vi "MTS_GenFileComment.vi"(0 "Resolution":dbl, 1 "Measurement Type":T2(ring)=enum."Image File", 3 "Parent File No":i32=-1, 5 "Pixels":i32[](array[numeric]), 7 "Info":string, 9 "Upper Left":T4, 11 "error in":errorcluster, 12 "Time Per Pixel [ms]":dbl, 13 "Trigger":dbl[](array[numeric])) -> (4 "Comment":string, 6 "Image Info":T3, 10 "Image Header":T1, 15 "error out":errorcluster)   [LabVIEW 2013]
panel:
  in  "Scan Axis":enum32{"x-y", "x-z", "y-x", "y-z", "z-x", "z-y"}(ring)
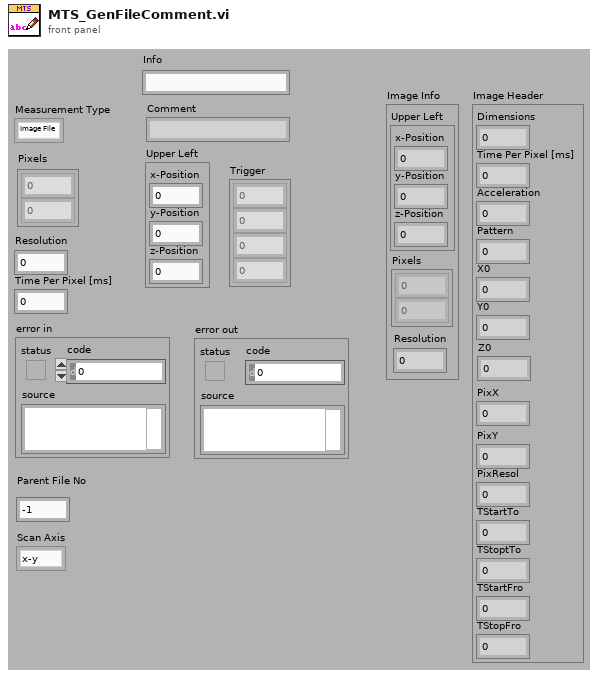
[diagram p1: front panel]
types:
  T1 = cluster{"Dimensions":i32, "Time Per Pixel [ms]":dbl, "Acceleration":i32, "Pattern":i32, "X0":sgl, "Y0":sgl, "Z0":dbl, "PixX":i32, "PixY":i32, "PixResol":sgl, "TStartTo":sgl, "TStoptTo":sgl, "TStartFro":sgl, "TStopFro":sgl}
  T2 = enum16{"not a pt3 File", "Image File", "Point Measurement", "Auto Point", "Line Scan", "Grid Scan"}
  T3 = cluster{"Upper Left":cluster{"x-Position":dbl, "y-Position":dbl, "z-Position":dbl}, "Pixels":i32[], "Resolution":dbl}
  T4 = cluster{"x-Position":dbl, "y-Position":dbl, "z-Position":dbl}
  T5 = enum16{"not a pt3 File", "Image File", "Point Measurement", "Auto Point"}
  T6 = cluster{"File No":i32, "File Path":path, "Parent File":i32, "File Type":enum16{"unknown", "pt3 File", "png Image", "bmp Image"}, "Measurement Type":enum16{"not a pt3 File", "Image File", "Point Measurement", "Auto Point", "Line Scan", "Grid Scan"}, "Upper Left":cluster{"x-Position":dbl, "y-Position":dbl, "z-Position":dbl}, "Pixels":i32[], "Scan Axis":enum32{"x-y", "x-z", "y-z"}, "Resolution":dbl, "PixelTime":dbl}
  T7 = cluster{"Trigger[0]":dbl, "Trigger[1]":dbl, "Trigger[2]":dbl, "Trigger[3]":dbl}
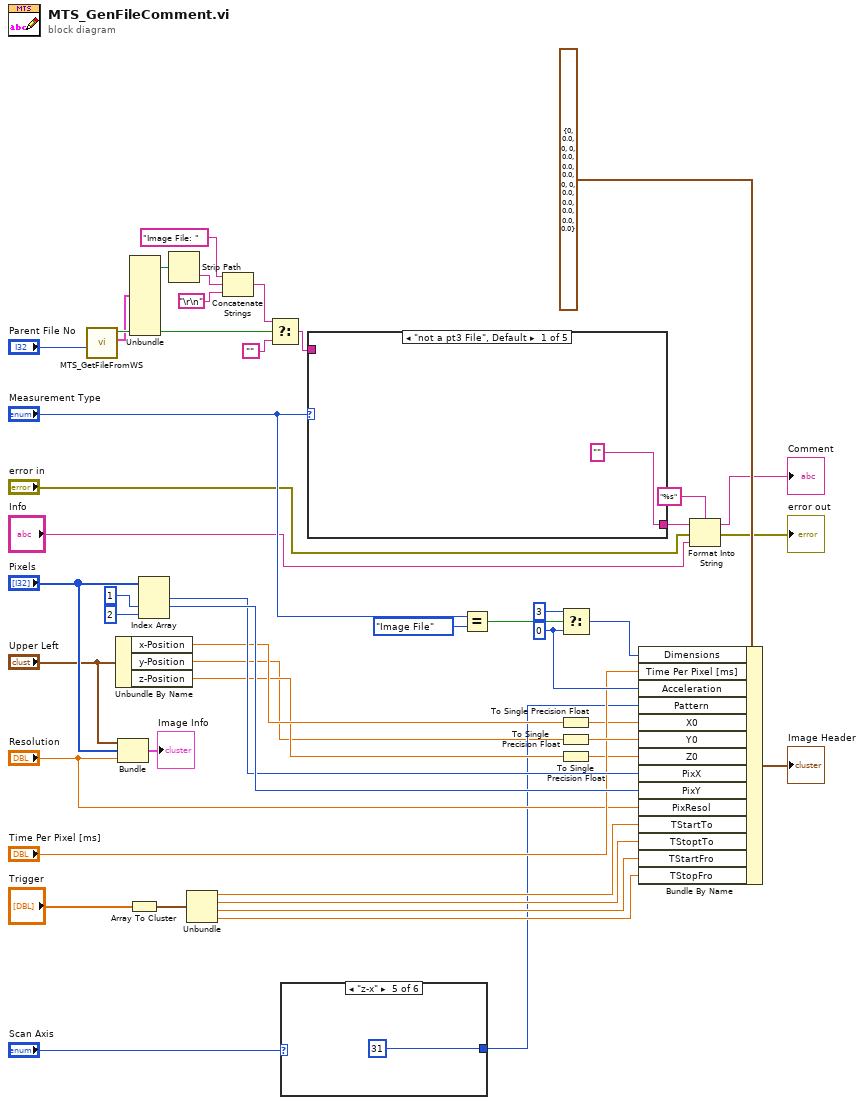
[diagram p0: block diagram]
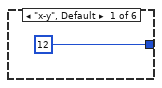
[diagram p2: hidden frame]
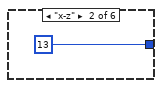
[diagram p3: hidden frame]
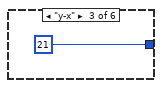
[diagram p4: hidden frame]
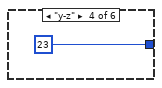
[diagram p5: hidden frame]
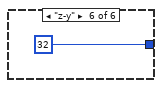
[diagram p6: hidden frame]
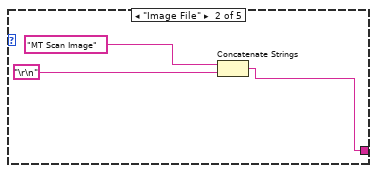
[diagram p7: hidden frame]
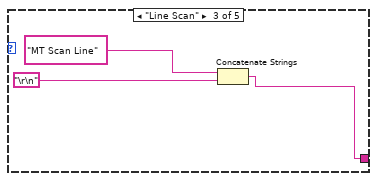
[diagram p8: hidden frame]
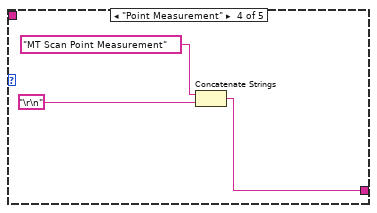
[diagram p9: hidden frame]
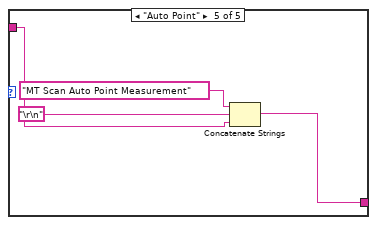
[diagram p10: hidden frame]
diagram:
  w38 = 0 ("f")
  n1 = call "MTS_GetFileFromWS.vi"("File No"="Parent File No") -> ("File Header"=w28:T6, "File Found"=w32:bool)  [unwired: 9 in]
  n2 = Unbundle By Name("Upper Left") -> ("x-Position"=w12:dbl, "y-Position"=w7:dbl, "z-Position"=w11:dbl)
  n3 = Bundle("Upper Left"="Upper Left", "Pixels"="Pixels", "Resolution"="Resolution") -> (→"Image Info":T3)  [unwired: 1 out]
  n4 = Array To Cluster(array="Trigger") -> (cluster=w18:T7)
  n5 = Unbundle(w28) -> ("File Path"=w27:path)  [unwired: 9 out]
  n6 = Index Array(array="Pixels", index #2=1 ("index"), index #3=2 ("index")) -> (element #1=w35:i32, element #2=w36:i32)  [unwired: 1 in, 1 out]
  n7 = Strip Path(path=w27) -> (name=w25:string)  [unwired: 1 out]
  n8 = Unbundle(w18) -> ("Trigger[0]"=w14:dbl, "Trigger[1]"=w17:dbl, "Trigger[2]"=w16:dbl, "Trigger[3]"=w15:dbl)
  n9 = Concatenate Strings("Image File: " ("string"), w25, "\r\n") -> (w26:string)
  n10 = Select(t=w26, s=w32, f="") -> (s? t:f=w30:string)
  n11 = case shown="\"z-x\"" "Scan Axis" {
    tunnel: [12 13 21 23 31 32] -> w8
    frame "x-y", Default {
    }
    frame "x-z" {
    }
    frame "y-x" {
    }
    frame "y-z" {
    }
    frame "z-x" {
    }
    frame "z-y" {
    }
  }
  n12 = case shown="\"not a pt3 File\", Default" "Measurement Type" {
    tunnel: w30 -> [_ _ _ _ w65]
    tunnel: ["" w55 w58 w61 w64] -> w5
    frame "not a pt3 File", Default {
    }
    frame "Image File" {
      n13 = Concatenate Strings("MT Scan Image" ("initial string"), "\r\n") -> (w55:string)
    }
    frame "Line Scan" {
      n14 = Concatenate Strings("MT Scan Line" ("initial string"), "\r\n") -> (w58:string)
    }
    frame "Point Measurement" {
      n15 = Concatenate Strings("MT Scan Point Measurement" ("initial string"), "\r\n") -> (w61:string)
    }
    frame "Auto Point" {
      n16 = Concatenate Strings("MT Scan Auto Point Measurement" ("initial string"), "\r\n", w65) -> (w64:string)
    }
  }
  n17 = Equal?(x="Measurement Type", y=T5."Image File") -> (x = y?=w41:bool)
  n18 = Select(t=3, s=w41, f=w38) -> (s? t:f=w39:i32)
  n19 = To Single Precision Float(number=w12) -> (single precision float=w13:sgl)
  n20 = To Single Precision Float(number=w7) -> (single precision float=w37:sgl)
  n21 = To Single Precision Float(number=w11) -> (single precision float=w10:sgl)
  n22 = Bundle By Name(cluster=T1 {"Dimensions"=0, "Time Per Pixel [ms]"=0.0, "Acceleration"=0, "Pattern"=0, "X0"=0.0, "Y0"=0.0, "Z0"=0.0, "PixX"=0, "PixY"=0, "PixResol"=0.0, "TStartTo"=0.0, "TStoptTo"=0.0, "TStartFro"=0.0, "TStopFro"=0.0} ("Image Header"), "Dimensions"=w39, "Time Per Pixel [ms]"="Time Per Pixel [ms]", "Acceleration"=w38, "Pattern"=w8, "X0"=w13, "Y0"=w37, "Z0"=w10, "PixX"=w35, "PixY"=w36, "PixResol"="Resolution", "TStartTo"=w14, "TStoptTo"=w17, "TStartFro"=w16, "TStopFro"=w15) -> (→"Image Header":T1)
  n23 = Format Into String(format string="%s", initial string=w5, error in="error in", "Info") -> (resulting string=→"Comment":string, error out=→"error out":errorcluster)
